vi "D.vi"(6 "G":string, 7 "5":string[](array[string]), 9 "C":string, 10 "F":string, 11 "A":string) -> (3 "D":string)   [LabVIEW 2017]
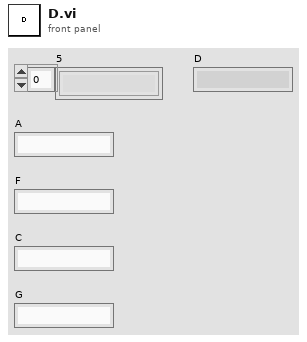
[diagram p1: front panel]
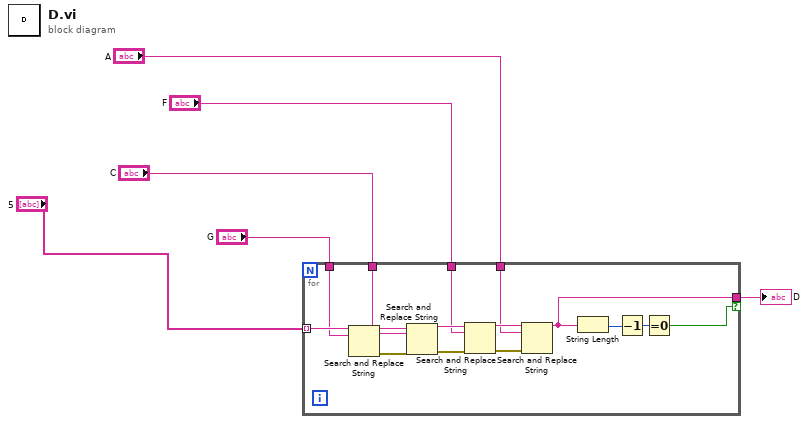
[diagram p0: block diagram]
diagram:
  n1 = for {
    tunnel: "5" -> [w21] mode=indexing
    tunnel: "G" -> [w14]
    tunnel: "C" -> [w13]
    tunnel: "F" -> [w12]
    tunnel: "A" -> [w11]
    tunnel: [w8] -> w6 if=w7
    n2 = Search and Replace String(input string=w21, search string=w14) -> (result string=w20:string, error out=w19:errorcluster)  [unwired: 6 in, 2 out]
    n3 = Search and Replace String(input string=w20, search string=w13, error in=w19) -> (result string=w18:string, error out=w17:errorcluster)  [unwired: 5 in, 2 out]
    n4 = Search and Replace String(input string=w18, search string=w12, error in=w17) -> (result string=w16:string, error out=w15:errorcluster)  [unwired: 5 in, 2 out]
    n5 = Search and Replace String(input string=w16, search string=w11, error in=w15) -> (result string=w8:string)  [unwired: 5 in, 3 out]
    n6 = String Length(string=w8) -> (length=w10:i32)
    n7 = Decrement(x=w10) -> (x-1=w9:i32)
    n8 = Equal To 0?(x=w9) -> (x = 0?=w7:bool)
  }
  "D" <- w6
